vi "Read Name.vi"(8 "error in (no error)":errorcluster, 11 "Platform Application":refnum<class "Platform Application.lvclass">) -> (0 "error out":errorcluster, 2 "Name":string, 3 "Platform Application out":refnum<class "Platform Application.lvclass">)   [LabVIEW 2015, in "NI_AWS_SNS.lvlib" / "Platform Application.lvclass"]
uses:
  Platform Application.lvclass
  Core/ARN/ARN.lvclass/ARN.ctl
  Core/ARN/Read ARN.vi
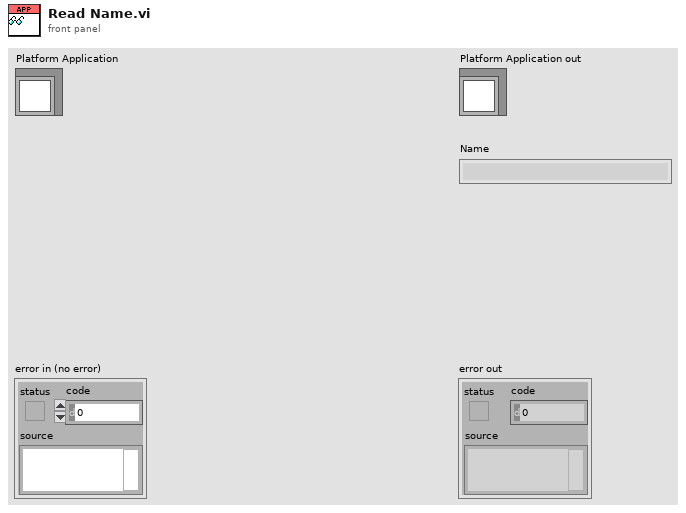
[diagram p1: front panel]
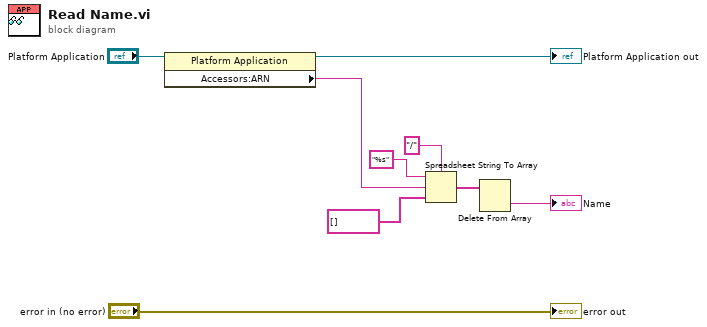
[diagram p0: block diagram]
diagram:
  n1 = property class="Platform Application"(reference="Platform Application") -> (reference out=→"Platform Application out":refnum<class "Platform Application.lvclass">, "Accessors:ARN"=w1:string)  [unwired: 1 in, 1 out]
  n2 = Spreadsheet String To Array(delimiter (Tab)="/", format string="%s", spreadsheet string=w1, array type (2D Dbl)=string[] []) -> (array=w4:string[])
  n3 = Delete From Array(array=w4) -> (deleted portion=→"Name":string)  [unwired: 2 in, 1 out]
  "error out" <- "error in (no error)"
